vi "CommandsInfo.vi"() -> ()   [LabVIEW 2014, in "examples.lvlib"]
uses:
  examples.lvlib
  vis/tango_vi.llb/tango.lvlib
panel:
  out "success":bool
  out "commands_info":T1(array[cluster])
  in  "device name":string="sys/tg_test/1"
  # "CommandInfo.level\n-----------------------\n\tOPERATOR = 0\n EXPERT = 1"
  # "CommandInfo.in-out-type\n-----------------------\n\tDEV_VOID = 0\n\tDEV_BOOLEAN = 1\n\tDEV_SHORT = 2\n\tDEV_LONG = 3\n\tDEV_FLOAT = 4\n\tDEV_DOUBLE = 5\n\tDEV_USHORT = 6\n\tDEV_ULONG = 7\n\tDEV_STRING = 8\n\tDEVVAR_CHARARRAY = 9\n\tDEVVAR_SHORTARRAY = 10\n\tDEVVAR_LONGARRAY = 11\n\tDEVVAR_FLOATARRAY = 12\n\tDEVVAR_DOUBLEARRAY = 13\n\tDEVVAR_USHORTARRAY = 14\n\tDEVVAR_ULONGARRAY = 15\n\tDEVVAR_STRINGARRAY = 16\n\tDEVVAR_LONGSTRINGARRAY = 17\n\tDEVVAR_DOUBLESTRINGARRAY = 18\n\tDEV_STATE = 19\n\tCONST_DEV_STRING = 20\n\tDEVVAR_BOOLEANARRAY = 21\n\tDEV_UCHAR = 22\n\tDEV_LONG64 = 23\n\tDEV_ULONG64 = 24\n\tDEVVAR_LONG64ARRAY = 25\n\tDEVVAR_ULONG64ARRAY = 26\n\tDEV_INT = 27\n\tDEV_ENCODED = 28"
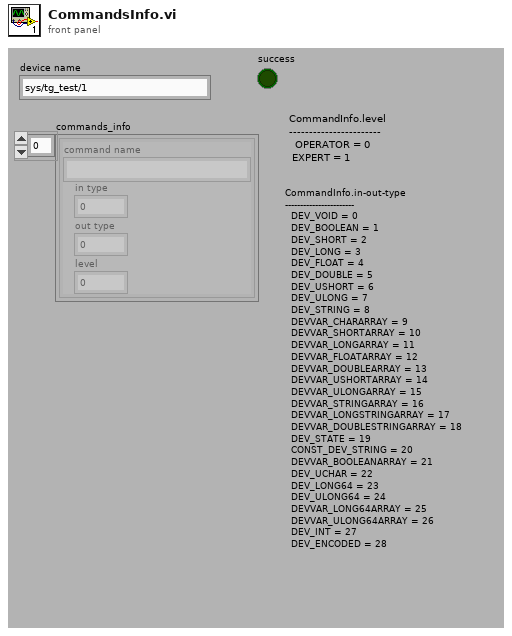
[diagram p1: front panel]
types:
  T1 = cluster{"command name":string, "in type":i16, "out type":i16, "level":i16}[]
  T2 = typedef "tango.lvlib/_CommandInfo_t.ctl" = cluster{"command name":string, "in Type":T3, "out Type":T3, "Tango Command Level":T4}
  T3 = typedef "tango.lvlib/_TangoDataType_t.ctl" = enum16{"VOID", "BOOLEAN", "SHORT", "LONG", "FLOAT", "DOUBLE", "USHORT", "ULONG", "STRING", "CHAR_ARRAY", "SHORT_ARRAY", "LONG_ARRAY", "FLOAT_ARRAY", "DOUBLE_ARRAY", "USHORT_ARRAY", "ULONG_ARRAY", "STRING_ARRAY", "LONG_STRING_ARRAY", "DOUBLE_STRING_ARRAY", "STATE", "CONST_STRING", "BOOLEAN_ARRAY", "UCHAR", "LONG64", "ULONG64", "LONG64_ARRAY", "ULONG64_ARRAY", "INT (not supported)", "ENCODED (not supported)", "ENUM", "PIPE_BLOB (not supported)", "STATE_ARRAY", "UNKNOW_DATA_TYPE"}
  T4 = typedef "tango.lvlib/_CommandLevel_t.ctl" = enum16{"OPERATOR", "EXPERT", "UNKNOWN_LEVEL"}
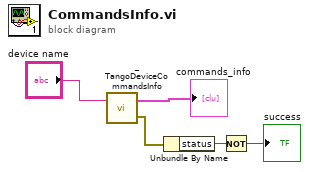
[diagram p0: block diagram]
diagram:
  n1 = call "_TangoDeviceCommandsInfo.vi"("device name"="device name") -> ("error out"=w3:errorcluster, "commands_info"=→"commands_info":T2[])  [unwired: 1 in]
  n2 = Unbundle By Name(w3) -> ("status"=w2:bool)
  n3 = Not(x=w2) -> (.not. x?=→"success":bool)
